vi "rpm nominali global.vi"() -> ()   [LabVIEW 2019]
panel:
  in  "rpm nominali":dbl
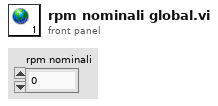
[diagram p1: front panel]
diagram:
